vi "PrimeNo.vi"() -> ()   [LabVIEW 2021]
panel:
  out "Result":string
  in  "Enter the No":i32
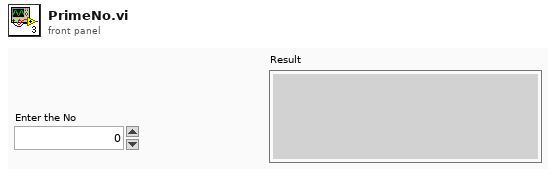
[diagram p1: front panel]
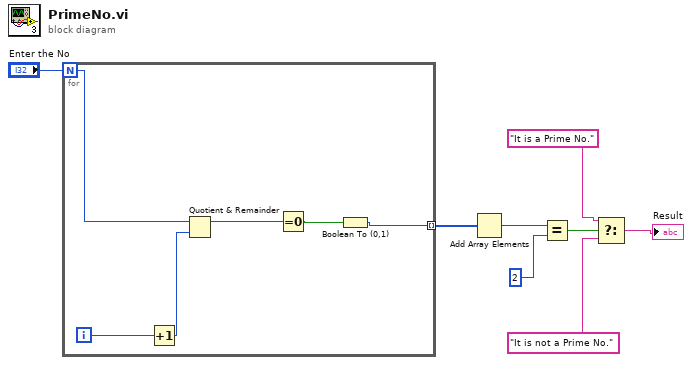
[diagram p0: block diagram]
diagram:
  n1 = for {
    N: "Enter the No" -> [w13]
    tunnel: [w9] -> w7 mode=indexing
    i -> [w14]
    n2 = Increment(x=w14) -> (x+1=w12:i32)
    n3 = Quotient & Remainder(x=w13, y=w12) -> (x-y*floor(x/y)=w11:i32)  [unwired: 1 out]
    n4 = Equal To 0?(x=w11) -> (x = 0?=w10:bool)
    n5 = Boolean To (0,1)(Boolean=w10) -> (0, 1=w9:i16)
  }
  n6 = Add Array Elements(numeric array=w7) -> (sum=w6:i16)
  n7 = Equal?(x=w6, y=i16 2) -> (x = y?=w4:bool)
  n8 = Select(t="It is a Prime No.", s=w4, f="It is not a Prime No.") -> (s? t:f=→"Result":string)
